vi "expressHeaderParser.vi"(11 "Header":string) -> (3 "Status code":i32)   [LabVIEW 2011]
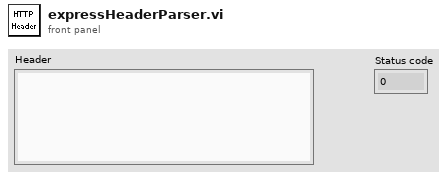
[diagram p1: front panel]
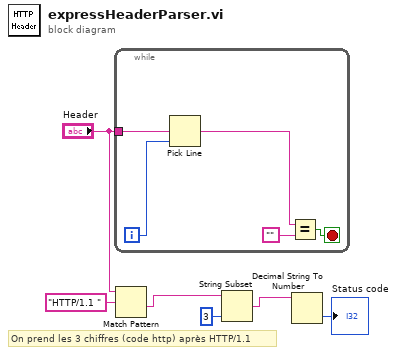
[diagram p0: block diagram]
diagram:
  # "On prend les 3 chiffres (code http) après HTTP/1.1"
  n1 = while {
    tunnel: "Header" -> [w11]
    i -> [w10]
    stop <- w9 stop-if-true
    n2 = Pick Line(multi-line string=w11, line index=w10) -> (output string=w8:string)  [unwired: 1 in]
    n3 = Equal?(x=w8, y="") -> (x = y?=w9:bool)
  }
  n4 = Match Pattern(string="Header", regular expression="HTTP/1.1 ") -> (after substring=w4:string)  [unwired: 1 in, 3 out]
  n5 = String Subset(string=w4, length (rest)=3 ("length (rest)")) -> (substring=w2:string)  [unwired: 1 in]
  n6 = Decimal String To Number(string=w2) -> (number=→"Status code":i32)  [unwired: 2 in, 1 out]
